vi "Select Channels.vi"(11 "Channels":i32[](array[numeric])=[0, 1, 2, 3, 4, 5, 6, 7]) -> (0 "Channels in Use":u32 format="%016b")   [LabVIEW 2013]
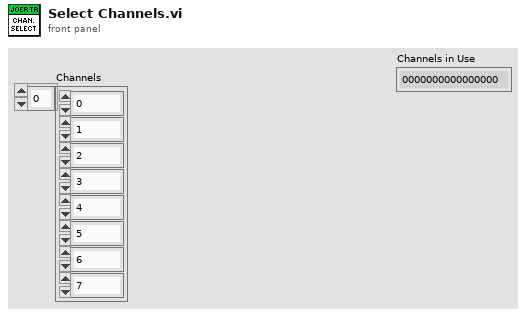
[diagram p1: front panel]
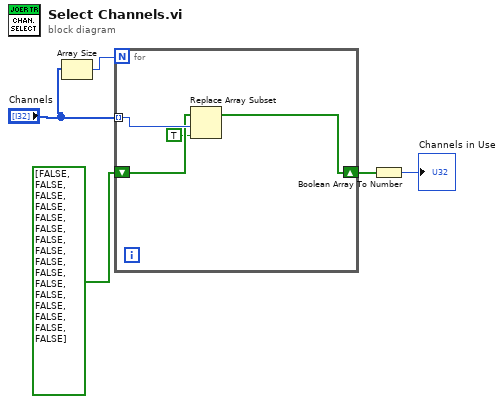
[diagram p0: block diagram]
diagram:
  n1 = Array Size(array="Channels") -> (size(s)=w1:i32)
  n2 = for {
    N: w1 -> [_]
    tunnel: "Channels" -> [w9] mode=indexing
    shift-right: [w6] -> w4
    shift-left: bool[] [FALSE, FALSE, FALSE, FALSE, FALSE, FALSE, FALSE, FALSE, FALSE, FALSE, FALSE, FALSE, FALSE, FALSE, FALSE, FALSE] -> [w8]
    n3 = Replace Array Subset(array=w8, new element=TRUE ("new element/subarray"), index=w9) -> (w6:bool[])
  }
  n4 = Boolean Array To Number(Boolean array=w4) -> (number=→"Channels in Use":u32)
